vi "SpecAn TxP Configure.vi"(0 "Instrument Handle In":refnum<k21>, 1 "Selector String":string, 5 "TxP Config":T1={"Measurement Interval (s)"=0.001, "RBW (Hz)"=20000000.0, "RBW Filter Type"=1, "RRC Alpha"=30000.0, "Averaging Enabled"=0, "Averaging Count"=10, "Averaging Type"=0} {"Averaging Type" items=["RMS", "Log", "Scalar", "Max", "Min"]; "Averaging Enabled" items=["False", "True"]; "RRC Alpha" format="%.3g"; "RBW Filter Type" items=["None"=5, "Gaussian"=1, "Flat"=2, "RRC"=6]; "RBW (Hz)" format="%.3p"; "Measurement Interval (s)" format="%.2p"}, 11 "error in (no error)":errorcluster) -> (4 "Instrument Handle Out":refnum<k21>, 15 "error out":errorcluster)   [LabVIEW 2016, in "RFmxSpecAn.lvlib"]
uses:
  RFmxSpecAn.lvlib
  Typedefs/SpecAn TxP Configuration.ctl
  <resource>/objmgr/RFmxSpecAn.rc
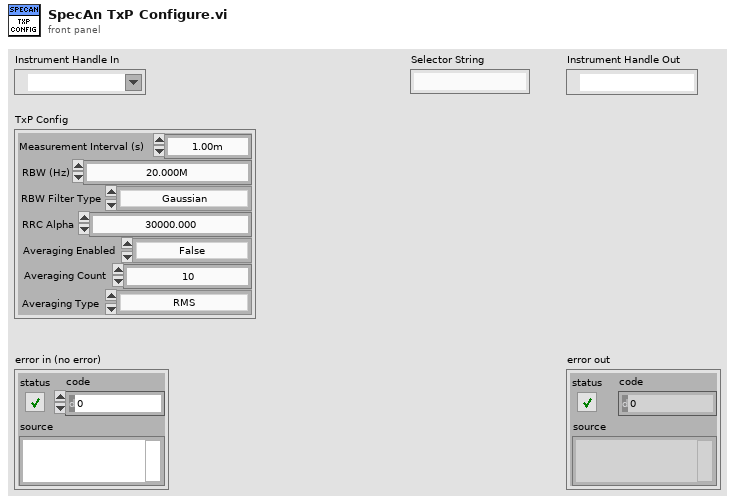
[diagram p1: front panel]
types:
  T1 = typedef "RFmxSpecAn.lvlib/SpecAn TxP Configuration.ctl" = cluster{"Measurement Interval (s)":dbl, "RBW (Hz)":dbl, "RBW Filter Type":i32, "RRC Alpha":dbl, "Averaging Enabled":i32, "Averaging Count":i32, "Averaging Type":i32}
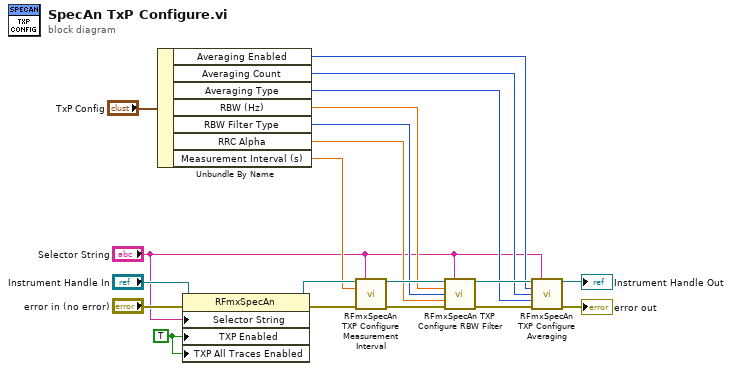
[diagram p0: block diagram]
diagram:
  w1 = TRUE ("TXP All Traces Enabled")
  n1 = Unbundle By Name("TxP Config") -> ("Averaging Enabled"=w3:i32, "Averaging Count"=w4:i32, "Averaging Type"=w5:i32, "RBW (Hz)"=w6:dbl, "RBW Filter Type"=w7:i32, "RRC Alpha"=w8:dbl, "Measurement Interval (s)"=w9:dbl)
  n2 = property class="RFmxSpecAn"(reference="Instrument Handle In", error in="error in (no error)", "Selector String"="Selector String", "TXP Enabled"=w1, "TXP All Traces Enabled"=w1) -> (reference out=w12:refnum<k21>, error out=w20:errorcluster)
  n3 = call <vilib>:"RFmxSpecAn TXP Configure Measurement Interval.vi"("Instrument Handle In"=w12, "Selector String"="Selector String", "Measurement Interval (s)"=w9, "error in (no error)"=w20) -> ("Instrument Handle Out"=w19:refnum<k21>, "error out"=w18:errorcluster)  [unwired: 10 in]
  n4 = call <vilib>:"RFmxSpecAn TXP Configure RBW Filter.vi"("Instrument Handle In"=w19, "Selector String"="Selector String", "RBW (Hz)"=w6, "RBW Filter Type"=w7, "RRC Alpha"=w8, "error in (no error)"=w18) -> ("Instrument Handle Out"=w16:refnum<k21>, "error out"=w17:errorcluster)  [unwired: 8 in]
  n5 = call <vilib>:"RFmxSpecAn TXP Configure Averaging.vi"("Instrument Handle In"=w16, "Selector String"="Selector String", "Averaging Enabled"=w3, "Averaging Count"=w4, "Averaging Type"=w5, "error in (no error)"=w17) -> ("Instrument Handle Out"=→"Instrument Handle Out":refnum<k21>, "error out"=→"error out":errorcluster)  [unwired: 8 in]
